vi "CFG Convert String to DAQmx Channel.vi"(5 "DAQ String":string) -> (2 "DAQmx Channel Input":tag)   [LabVIEW 2012]
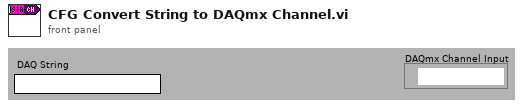
[diagram p1: front panel]
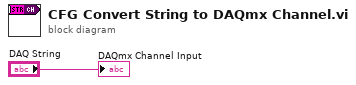
[diagram p0: block diagram]
diagram:
  "DAQmx Channel Input" <- "DAQ String"
